vi "Edit_Server_Channel.vi"(5 "Mode":T1(ring)) -> ()   [LabVIEW 2016]
uses:
  Sub VIs/ADAM Controls/Ch_description_ADAM.ctl
  Sub VIs/ADAM Controls/Module_type_ADAM.ctl
  Sub VIs/ADAM Controls/Function_ADAM.ctl
  Sub VIs/ADAM Controls/Channel_State.ctl
  Sub VIs/ADAM Controls/Calib_type_ADAM.ctl
  Sub VIs/ADAM Controls/Address.ctl
  Sub VIs/ADAM Controls/Channel_names.ctl
panel:
  out "Message":string
  in  "Value":dbl
  out "String":string
  out "Help":string
  in  "Search String":string
  in  "Channel Names":i32(listbox)
  in  "Ch Description":T2={"Ch Name"="", "Type"="", "Function"=enum."Analogue Input", "Ch State"=enum."On", "Calibration type"="", "A"=0.0, "B"=0.0, "C"=0.0, "D"=0.0, "Comments"="", "Address"={"Main"=0, "Ch."=0, "Sub"=0, "Port Name"=""}, "String"="", "Duty"=65535} {"Duty" format="%016b"; "D" format="%#_5g"; "C" format="%#_5g"; "B" format="%#_5g"; "A" format="%#_5g"}
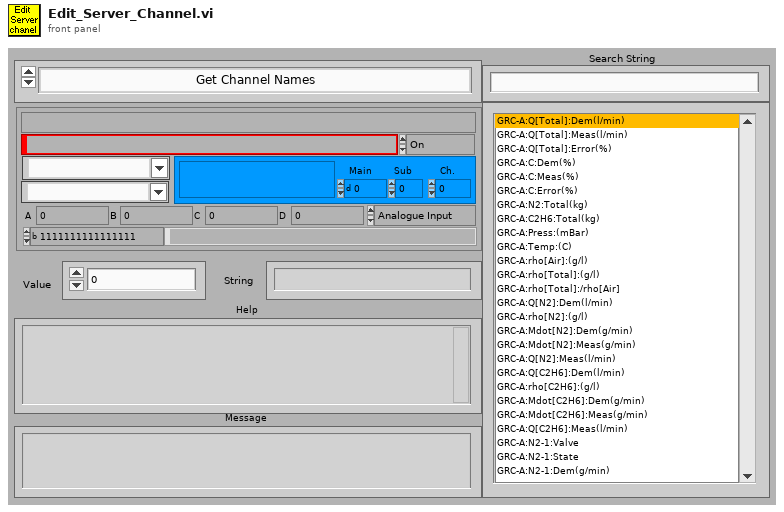
[diagram p1: front panel]
types:
  T1 = enum16{"Get Channel Names", "Get Current Value", "Update Channel Value", "Update Channel Description"}
  T2 = typedef "Ch_description_ADAM.ctl" = cluster{"Ch Name":string, "Type":T3, "Function":T4, "Ch State":T5, "Calibration type":T6, "A":dbl, "B":dbl, "C":dbl, "D":dbl, "Comments":string, "Address":T7, "String":string, "Duty":u16}
  T3 = typedef "Module_type_ADAM.ctl" = string
  T4 = typedef "Function_ADAM.ctl" = enum16{"Analogue Input", "Digital Input", "Event counter", "Event rate", "Analogue Output", "Digital Output", "Relay Output"}
  T5 = typedef "Channel_State.ctl" = enum16{"On", "Off", "Always On", "Always Off"}
  T6 = typedef "Calib_type_ADAM.ctl" = string
  T7 = typedef "Address.ctl" = cluster{"Main":i32, "Ch.":i32, "Sub":i32, "Port Name":string}
  T8 = typedef "Channel_names.ctl" = enum16{"Active Only", "Active + Off", "All Channels"}
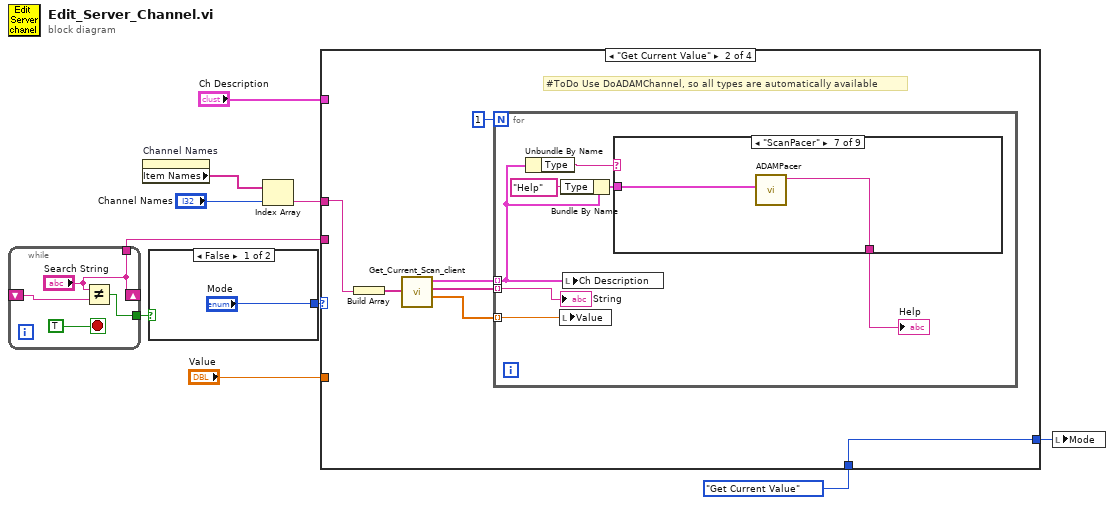
[diagram p0: block diagram]
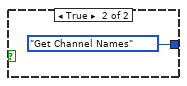
[diagram p2: hidden frame]
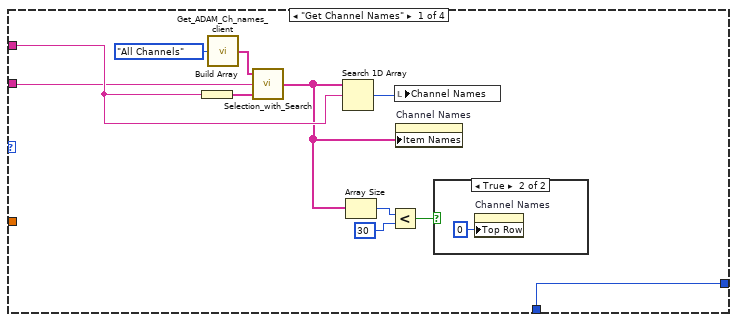
[diagram p3: hidden frame]
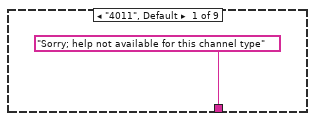
[diagram p5: hidden frame]
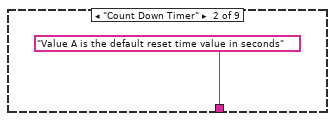
[diagram p6: hidden frame]
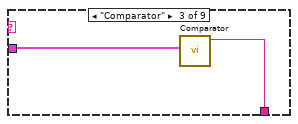
[diagram p7: hidden frame]
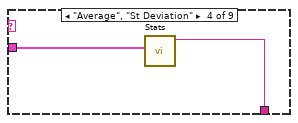
[diagram p8: hidden frame]
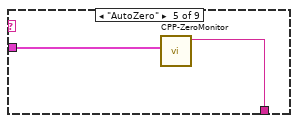
[diagram p9: hidden frame]
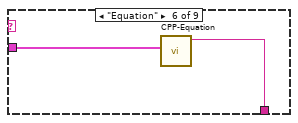
[diagram p10: hidden frame]
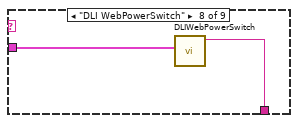
[diagram p11: hidden frame]
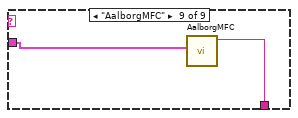
[diagram p12: hidden frame]
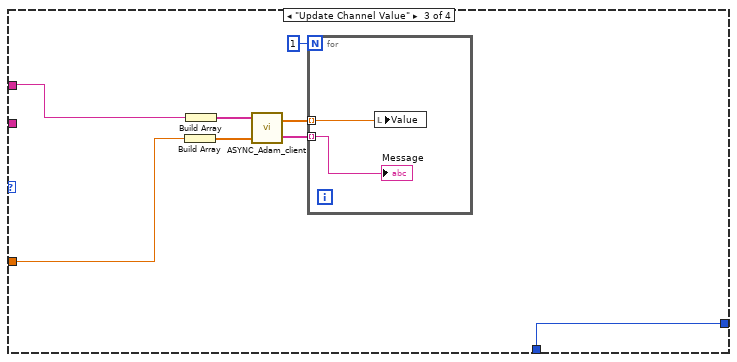
[diagram p13: hidden frame]
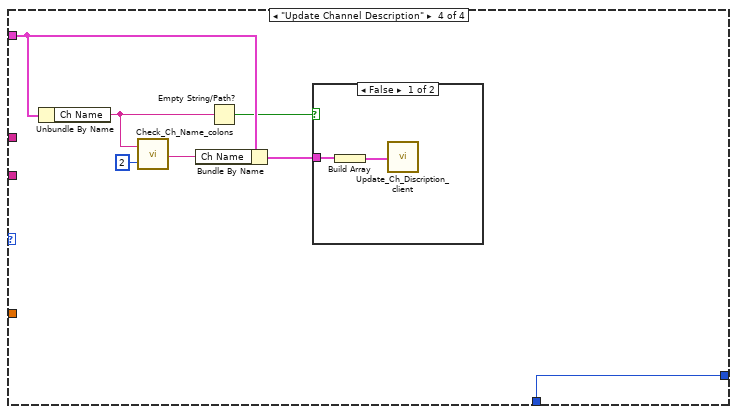
[diagram p14: hidden frame]
diagram:
  n1 = while {
    shift-right: ["Search String"] -> _
    shift-left: _ -> [w14]
    tunnel: [w13] -> w3
    tunnel: ["Search String"] -> w2
    stop <- TRUE stop-if-true
    n2 = Not Equal?(x="Search String", y=w14) -> (x != y?=w13:bool)
  }
  n3 = property on="Channel Names" class="LstBox (strict)"() -> ("Item Names"=w8:string[])  [unwired: 2 in, 2 out]
  n4 = case shown="False" w3 {
    tunnel: ["Mode" T1."Get Channel Names" ("Mode")] -> w10
    frame False {
    }
    frame True {
    }
  }
  n5 = Index Array(array=w8, index="Channel Names") -> (element=w7:string)
  n6 = case shown="\"Get Current Value\"" w10 {
    tunnel: w7 -> [w23 w34 w66 _]
    tunnel: "Value" -> [_ _ w63 _]
    tunnel: "Ch Description" -> [_ _ _ w74]
    tunnel: T1."Get Current Value" ("Mode") -> [w26 w29 w59 w75]
    tunnel: [w26 w29 w59 w75] -> w4
    tunnel: w2 -> [w21 _ _ _]
    frame "Get Channel Names" {
      n7 = Build Array(w23) -> (w24:string[])
      n8 = call "Get_ADAM_Ch_names_client.vi"("Channel names set"=Channel_names."All Channels") -> ("Ch names"=w25:string[])
      n9 = call "Selection_with_Search.vi"("Selected Channel Names"=w24, "Search String"=w21, "All Channel Names"=w25) -> ("Item Names"=w20:string[])
      n10 = Search 1D Array(1D array=w20, element=w23) -> (index of element=w22:i32)  [unwired: 1 out]
      n11 = Array Size(array=w20) -> (size(s)=w19:i32)
      n12 = Less?(x=w19, y=30) -> (x < y?=w17:bool)
      n13 = local write "Channel Names"(w22) -> ()
      n14 = property on="Channel Names" class="LstBox (strict)"("Item Names"=w20) -> ()  [unwired: 2 in, 2 out]
      n15 = case shown="True" w17 {
        frame False {
        }
        frame True {
          n16 = property on="Channel Names" class="LstBox (strict)"("Top Row"=0) -> ()  [unwired: 2 in, 2 out]
        }
      }
    }
    frame "Get Current Value" {
      # "#ToDo Use DoADAMChannel, so all types are automatically available"
      n17 = Build Array(w34) -> (w35:string[])
      n18 = call "Get_Current_Scan_client.vi"("ADAM Ch Names"=w35) -> ("Ch Description Array"=w32:T2[], "String values"=w31:string[], "Numerical Values"=w30:dbl[])  [unwired: 1 out]
      n19 = for {
        N: 1 -> [_]
        tunnel: w32 -> [w40] mode=indexing
        tunnel: w31 -> [w37] mode=indexing
        tunnel: w30 -> [w36] mode=indexing
        n20 = Unbundle By Name(w40) -> ("Type"=w42:T3)
        n21 = local write "Value"(w36) -> ()
        n22 = Bundle By Name(cluster=w40, "Type"=T3 "Help") -> (w39:T2)
        n23 = local write "Ch Description"(w40) -> ()
        n24 = case shown="\"ScanPacer\"" w42 {
          tunnel: ["Sorry; help not available for this channel type" "Value A is the default reset time value in seconds" w46 w47 w49 w51 w53 w55 w57] -> w38
          tunnel: w39 -> [_ _ w45 w48 w50 w52 w54 w56 w58]
          frame "4011", Default {
          }
          frame "Count Down Timer" {
          }
          frame "Comparator" {
            n25 = call "Comparator.vi"("Ch Description"=w45) -> ("HelpText"=w46:string)  [unwired: 6 in, 2 out]
          }
          frame "Average", "St Deviation" {
            n26 = call "Stats.vi"("Ch Description"=w48) -> ("HelpText"=w47:string)  [unwired: 6 in, 2 out]
          }
          frame "AutoZero" {
            n27 = call "CPP-ZeroMonitor.vi"("Ch Description"=w50) -> ("HelpText"=w49:string)  [unwired: 6 in, 2 out]
          }
          frame "Equation" {
            n28 = call "CPP-Equation.vi"("Ch Description"=w52) -> ("HelpText"=w51:string)  [unwired: 6 in, 2 out]
          }
          frame "ScanPacer" {
            n29 = call "ADAMPacer.vi"("Ch Description"=w54) -> ("HelpText"=w53:string)  [unwired: 6 in, 2 out]
          }
          frame "DLI WebPowerSwitch" {
            n30 = call "DLIWebPowerSwitch.vi"("Ch Description"=w56) -> ("HelpText"=w55:string)  [unwired: 6 in, 2 out]
          }
          frame "AalborgMFC" {
            n31 = call "AalborgMFC.vi"("Ch Description"=w58) -> ("HelpText"=w57:string)  [unwired: 6 in, 2 out]
          }
        }
        "Help" <- w38
        "String" <- w37
      }
    }
    frame "Update Channel Value" {
      n32 = Build Array(w63) -> (w64:dbl[])
      n33 = Build Array(w66) -> (w65:string[])
      n34 = call "ASYNC_Adam_client.vi"("Values"=w64, "Channel Names"=w65) -> ("Scan Comments"=w60:string[], "Calibrated Units"=w61:dbl[])  [unwired: 1 in]
      n35 = for {
        N: 1 -> [_]
        tunnel: w61 -> [w68] mode=indexing
        tunnel: w60 -> [w67] mode=indexing
        n36 = local write "Value"(w68) -> ()
        "Message" <- w67
      }
    }
    frame "Update Channel Description" {
      n37 = Unbundle By Name(w74) -> ("Ch Name"=w73:string)
      n38 = call "Check_Ch_Name_colons.vi"("No of Colons"=2, "Ch Name in"=w73) -> ("Ch Name out"=w71:string)
      n39 = Bundle By Name(cluster=w74, "Ch Name"=w71) -> (w70:T2)
      n40 = Empty String/Path?(string/path=w73) -> (empty?=w69:bool)
      n41 = case shown="False" w69 {
        tunnel: w70 -> [w76 _]
        frame False {
          n42 = Build Array(w76) -> (w77:T2[])
          n43 = call "Update_Ch_Discription_client.vi"("Channels to update In"=w77) -> ()  [unwired: 1 out]
        }
        frame True {
        }
      }
    }
  }
  n44 = local write "Mode"(w4) -> ()
